vi "Calculate Vertex Array.vi"(8 "error in (no error)":errorcluster, 10 "2D Error Bar Datatype.lvclass in":refnum<class "2D Error Bar Datatype.lvclass">, 11 "Plot Representation In":T1) -> (0 "error out":errorcluster, 2 "2D Error Bar Datatype.lvclass out":refnum<class "2D Error Bar Datatype.lvclass">, 3 "Plot Representation Out":T1)   [LabVIEW 2017, in "2D Error Bar Datatype.lvclass"]
uses:
  <vilib>/Math Plots/2D Math Plots/2D Error Bar/2D Error Bar Datatype/2D Error Bar Datatype.lvclass
  <vilib>/Math Plots/2D Math Plots/2D Plot/2D Plot/Typedef/Plot Representation.ctl
  <vilib>/Math Plots/2D Math Plots/2D Plot/2D Plot/Typedef/Range Cluster.ctl
  <vilib>/Math Plots/2D Math Plots/2D Error Bar/2D Error Bar Datatype/2D Error Bar Datatype.lvclass/2D Error Bar Datatype.ctl
  <vilib>/Math Plots/2D Math Plots/2D Plot/2D Plot/2D Plot.lvclass
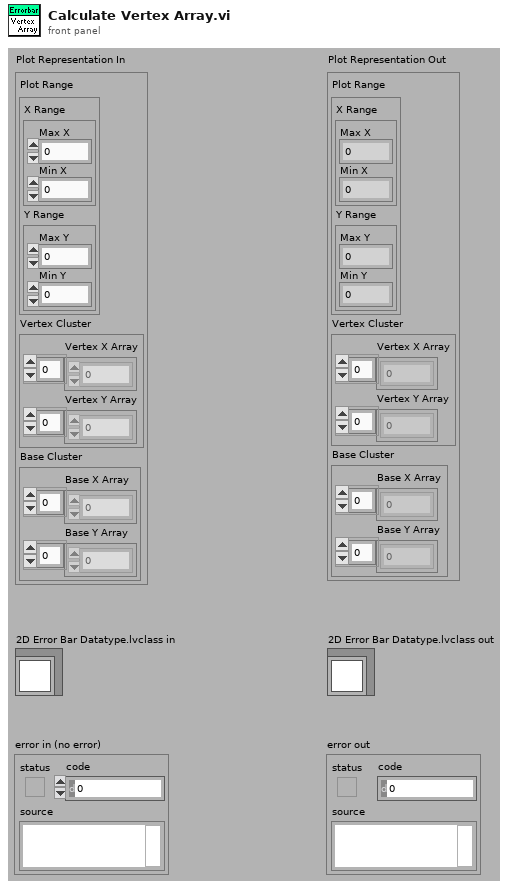
[diagram p1: front panel]
types:
  T1 = typedef "2D Plot.lvclass/Plot Representation.ctl" = cluster{"Plot Range":T2, "Vertex Cluster":cluster{"Vertex X Array":dbl[], "Vertex Y Array":dbl[]}, "Base Cluster":cluster{"Base X Array":dbl[], "Base Y Array":dbl[]}}
  T2 = typedef "2D Plot.lvclass/Range Cluster.ctl" = cluster{"X Range":cluster{"Max X":dbl, "Min X":dbl}, "Y Range":cluster{"Max Y":dbl, "Min Y":dbl}}
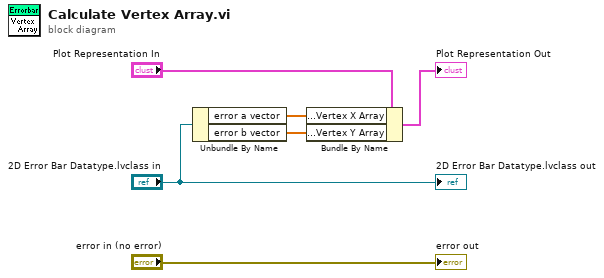
[diagram p0: block diagram]
diagram:
  n1 = Unbundle By Name("2D Error Bar Datatype.lvclass in") -> ("error a vector"=w2:dbl[], "error b vector"=w1:dbl[])
  n2 = Bundle By Name(cluster="Plot Representation In", "Vertex Cluster.Vertex X Array"=w2, "Vertex Cluster.Vertex Y Array"=w1) -> (→"Plot Representation Out":T1)
  "2D Error Bar Datatype.lvclass out" <- "2D Error Bar Datatype.lvclass in"
  "error out" <- "error in (no error)"
